vi "Create Feed.vi"(0 "Packages Path":path, 11 "error in (no error)":errorcluster) -> (15 "error out":errorcluster)   [LabVIEW 2021, in "Packager Helpers.lvlib"]
uses:
  Packager Helpers.lvlib
  Path Functions/Path Functions.lvlib
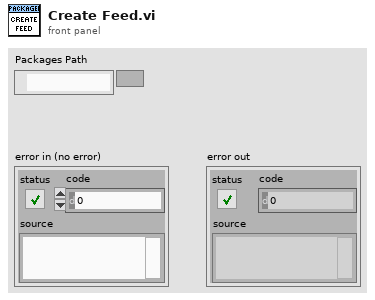
[diagram p1: front panel]
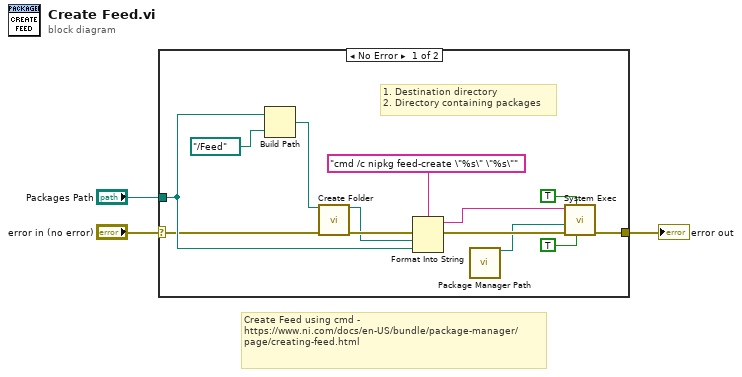
[diagram p0: block diagram]
diagram:
  # "Create Feed using cmd -\nhttps://www.ni.com/docs/en-US/bundle/package-manager/page/creating-feed.html"
  n1 = case shown="No Error" "error in (no error)" {
    selector: "error in (no error)" -> [w13 w17]
    tunnel: "Packages Path" -> [w15 _]
    tunnel: [w6 w17] -> w1
    frame No Error {
      # "1. Destination directory\n2. Directory containing packages"
      n2 = Build Path(base path=w15, name or relative path=path "../Feed") -> (appended path=w14:path)
      n3 = call "Create Folder.vi"("Directory Path"=w14, "error in (no error)"=w13) -> ("Dup Directory Path"=w11:path, "error out"=w12:errorcluster)  [unwired: 12 in]
      n4 = Format Into String(format string="cmd /c nipkg feed-create \"%s\" \"%s\"", error in=w12, w11, w15) -> (resulting string=w9:string, error out=w10:errorcluster)  [unwired: 1 in]
      n5 = call "Package Manager Path.vi"() -> ("Package Manager Path"=w4:path)  [unwired: 15 in]
      n6 = call <vilib>:"System Exec.vi"("run minimized? (F)"=TRUE, "wait until completion? (T)"=TRUE, "error in (no error)"=w10, "working directory"=w4, "command line"=w9) -> ("error out"=w6:errorcluster)  [unwired: 3 in, 3 out]
    }
    frame Error {
    }
  }
  "error out" <- w1
